vi "Template Main.vi"(8 "error in (no error)":errorcluster) -> (0 "error out":errorcluster)   [LabVIEW 2020, in "Module Template.lvlib"]
doc: "This template is for the Modules in the Project."
uses:
  Module Template.lvlib
  Private Controls/FG Actions.ctl
  Private Controls/Module Data.ctl
  Private Controls/Message Cluster.ctl
  Private Controls/Message enum.ctl
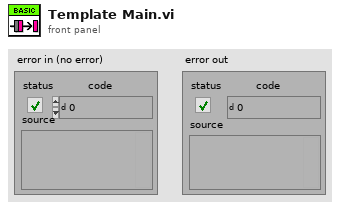
[diagram p1: front panel]
types:
  T1 = typedef "Module Template.lvlib/Module Data.ctl" = cluster{"Data":variant}
  T2 = typedef "Module Template.lvlib/FG Actions.ctl" = enum16{"Get", "Set", "Clear"}
  T3 = typedef "Module Template.lvlib/Message Cluster.ctl" = cluster{"Message":T4, "Data":variant}
  T4 = typedef "Module Template.lvlib/Message enum.ctl" = enum16{"Initialize", "State", "Error", "Exit"}
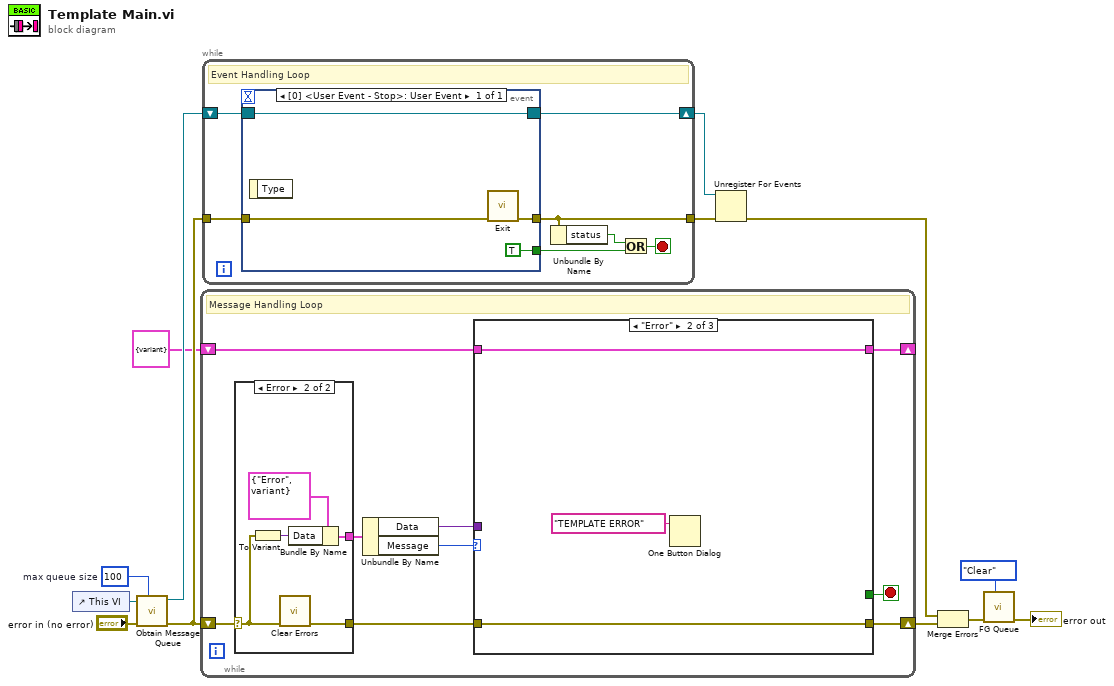
[diagram p0: block diagram]
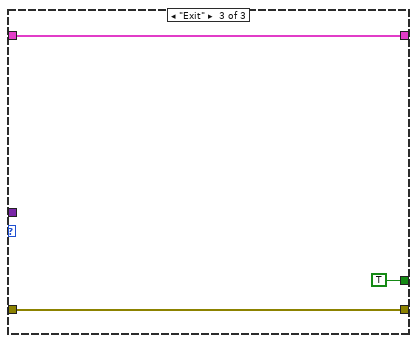
[diagram p3: hidden frame]
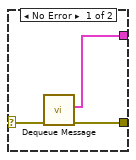
[diagram p4: hidden frame]
diagram:
  w7 = 100  # max queue size
  n1 = control-ref of="This VI"() -> (w8:refnum<vi>)
  n2 = call "Obtain Message Queue.vi"("max queue size (-1, unlimited)"=w7, "error in (no error)"="error in (no error)", "VI Reference"=w8) -> ("error out"=w3:errorcluster, "Event Registration Refnum"=w10:refnum<event-registration>)  [unwired: 7 in]
  n3 = while {
    shift-right: [w17] -> w13
    shift-left: w3 -> [w22]
    shift-right: [w14] -> _
    shift-left: T1 {"Data"=variant} ("Message Cluster") -> [w15]
    stop <- w16 stop-if-true
    # "Message Handling Loop"
    n4 = case shown="Error" w22 {
      selector: w22 -> [w31 w37]
      tunnel: [w32 w38] -> w18
      tunnel: [w33 w34] -> w21
      frame No Error {
        n5 = call "Dequeue Message.vi"("error in (no error)"=w31) -> ("error out"=w32:errorcluster, "Element"=w33:T3)  [unwired: 9 in]
      }
      frame Error {
        n6 = To Variant(anything=w37) -> (Variant=w35:variant)
        n7 = call <vilib>:"Clear Errors.vi"("error in (no error)"=w37) -> ("error out"=w38:errorcluster)  [unwired: 5 in, 1 out]
        n8 = Bundle By Name(cluster=T3 {"Message"=enum."Error", "Data"=variant} ("Message Cluster"), "Data"=w35) -> (w34:T3)
      }
    }
    n9 = Unbundle By Name(w21) -> ("Data"=w19:variant, "Message"=w20:T4)
    n10 = case shown="\"Error\"" w20 {
      tunnel: w19 -> [_ _ _]
      tunnel: w18 -> [w24 w27 w30]
      tunnel: [w24 w27 w30] -> w17
      tunnel: [_ _ TRUE] -> w16
      tunnel: w15 -> [w23 w25 w28]
      tunnel: [w23 w25 w28] -> w14
      frame "Initialize", Default {
      }
      frame "Error" {
        n11 = One Button Dialog(message="TEMPLATE ERROR") -> ()  [unwired: 1 in, 1 out]
      }
      frame "Exit" {
      }
    }
  }
  n12 = while {
    shift-right: [w44] -> w11
    shift-left: w10 -> [w45]
    tunnel: w3 -> [w42]
    tunnel: [w40] -> w2
    stop <- w41 stop-if-true
    # "Event Handling Loop"
    n13 = event shown="[0] <User Event - Stop>: User Event" {
      selector: w45 -> [w46]
      dyn-events: [w46] -> w44
      timeout: _ -> [_]
      tunnel: [TRUE ("Discard?")] -> w43
      tunnel: w42 -> [w48]
      tunnel: [w47] -> w40
      event User Event {
        n14 = event-data() -> ()  [unwired: 1 in, 1 out]
        n15 = call "Exit.vi"("error in (no error)"=w48) -> ("error out"=w47:errorcluster)  [unwired: 10 in]
      }
    }
    n16 = Unbundle By Name(w40) -> ("status"=w39:bool)
    n17 = Or(x=w39, y=w43) -> (x .or. y?=w41:bool)
  }
  n18 = Unregister For Events(event registration refnum=w11, error in=w2) -> (error out=w12:errorcluster)
  n19 = Merge Errors(w12, w13) -> (w5:errorcluster)
  n20 = call "FG Queue.vi"("FG Actions"=FG_Actions."Clear", "error in (no error)"=w5) -> ("error out"=→"error out":errorcluster)  [unwired: 8 in, 1 out]
